vi "Set parameters.vi"(8 "error in (no error)":errorcluster caption="entrée d'erreur (pas d'erreur)", 11 "OWIS_TANGO en entrée":refnum<class "OWIS_TANGO.lvclass">) -> (0 "error out":errorcluster caption="sortie d'erreur", 3 "OWIS_TANGO en sortie":refnum<class "OWIS_TANGO.lvclass">)   [LabVIEW 2020, in "OWIS_TANGO.lvclass"]
uses:
  OWIS_TANGO.lvclass
  C:/dev/TRANCON/Classes/GeneralFunctionality/GeneralFunctionality.lvclass
  C:/dev/TRANCON/Classes/Delay Line/DelayLine.lvclass
  GeneralFunctionality/GeneralFunctionality.lvclass/GeneralFunctionality.ctl
  DelayLineLS4/LS4_parameters.ctl
  Config/Config.lvclass
  DelayLine.lvclass
  GeneralFunctionality/GeneralFunctionality.lvclass
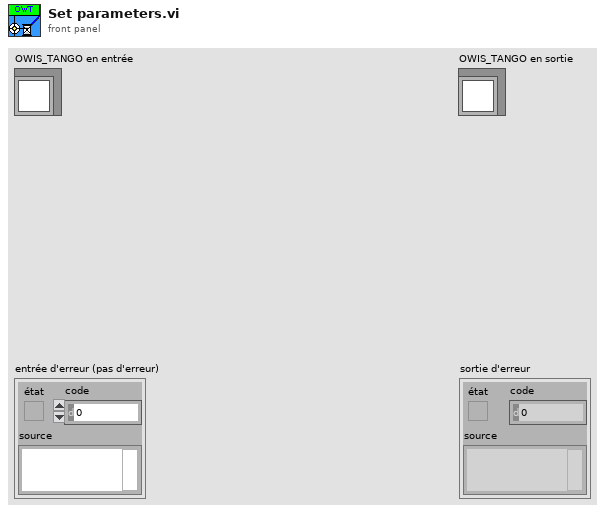
[diagram p1: front panel]
types:
  T1 = typedef "DelayLine.lvclass/LS4_parameters.ctl" = string
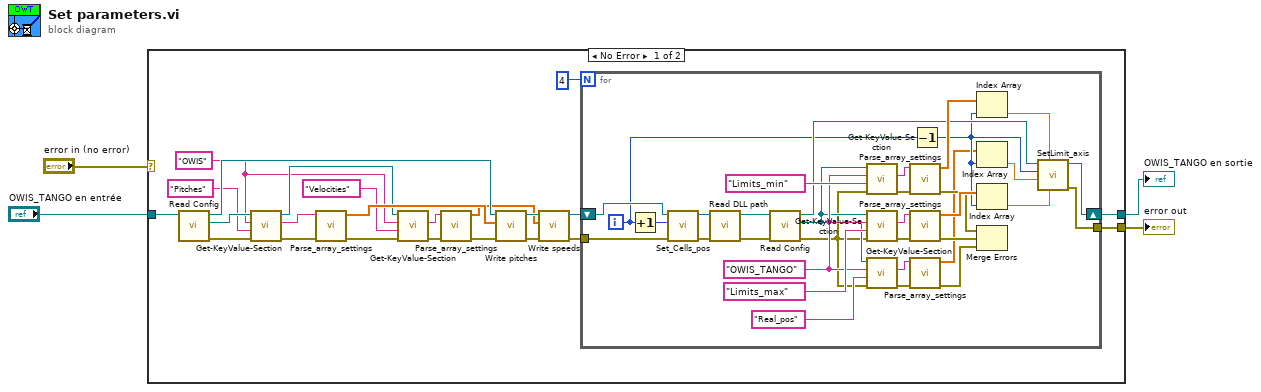
[diagram p0: block diagram]
diagram:
  n1 = case shown="No Error" "error in (no error)" {
    selector: "error in (no error)" -> [_ w62]
    tunnel: [w6 w61] -> w3
    tunnel: "OWIS_TANGO en entrée" -> [w23 w61]
    tunnel: [w7 w62] -> w1
    frame No Error {
      w10 = "OWIS" ("Section")
      n2 = call "Read Config.vi"("GeneralFunctionality en entrée"=w23) -> ("error out"=w19:errorcluster, "Config.lvclass"=w18:refnum<class "Config.lvclass">, "GeneralFunctionality en sortie"=w22:refnum<class "OWIS_TANGO.lvclass">)  [unwired: 8 in]
      n3 = call-dynamic "Get-KeyValue-Section.vi"("error in (no error)"=w19, "Key"="Pitches", "Section"=w10, "Config in"=w18) -> ("error out"=w16:errorcluster, "Value"=w15:string, "Config out"=w14:refnum<class "Config.lvclass">)  [unwired: 5 in]
      n4 = call "Parse_array_settings.vi"("error in (no error)"=w16, "Value"=w15) -> ("error out"=w13:errorcluster, "Array"=w21:dbl[])  [unwired: 8 in]
      n5 = call-dynamic "Get-KeyValue-Section.vi"("error in (no error)"=w13, "Key"="Velocities", "Section"=w10, "Config in"=w14) -> ("error out"=w12:errorcluster, "Value"=w11:string)  [unwired: 5 in, 1 out]
      n6 = call "Parse_array_settings.vi"("error in (no error)"=w12, "Value"=w11) -> ("error out"=w8:errorcluster, "Array"=w20:dbl[])  [unwired: 8 in]
      n7 = call-dynamic "Write pitches.vi"("error in (no error)"=w8, "pitches"=w21, "DelayLine in"=w22) -> ("error out"=w27:errorcluster, "DelayLine out"=w26:refnum<class "OWIS_TANGO.lvclass">)  [unwired: 7 in]
      n8 = call-dynamic "Write speeds.vi"("error in (no error)"=w27, "speeds"=w20, "DelayLine in"=w26) -> ("error out"=w25:errorcluster, "DelayLine out"=w24:refnum<class "OWIS_TANGO.lvclass">)  [unwired: 7 in]
      n9 = for {
        N: 4 -> [_]
        tunnel: w25 -> [w60]
        tunnel: [w33] -> w7
        shift-right: [w32] -> w6
        shift-left: w24 -> [w59]
        i -> [w28]
        w42 = "OWIS_TANGO" ("Section")
        n10 = Increment(x=w28) -> (x+1=w29:i32)
        n11 = call "Set_Cells_pos.vi"("error in (no error)"=w60, "axis"=w29, "DelayLine in"=w59) -> ("error out"=w30:errorcluster, "DelayLine out"=w31:refnum<class "OWIS_TANGO.lvclass">)  [unwired: 7 in]
        n12 = call "Read DLL path.vi"("error in (no error)"=w30, "DelayLine in"=w31) -> ("error out"=w55:errorcluster, "DelayLine out"=w47:refnum<class "OWIS_TANGO.lvclass">)  [unwired: 7 in, 1 out]
        n13 = call "Read Config.vi"("error in (no error)"=w55, "GeneralFunctionality en entrée"=w47) -> ("error out"=w40:errorcluster, "Config.lvclass"=w41:refnum<class "Config.lvclass">, "GeneralFunctionality en sortie"=w46:refnum<class "OWIS_TANGO.lvclass">)  [unwired: 7 in]
        n14 = call-dynamic "Get-KeyValue-Section.vi"("error in (no error)"=w40, "Key"=T1 "Limits_min" ("Section"), "Section"=w42, "Config in"=w41) -> ("error out"=w57:errorcluster, "Value"=w58:string)  [unwired: 5 in, 1 out]
        n15 = call-dynamic "Get-KeyValue-Section.vi"("error in (no error)"=w40, "Key"=T1 "Limits_max" ("Section"), "Section"=w42, "Config in"=w41) -> ("error out"=w53:errorcluster, "Value"=w52:string)  [unwired: 5 in, 1 out]
        n16 = call-dynamic "Get-KeyValue-Section.vi"("error in (no error)"=w40, "Key"="Real_pos", "Section"=w42, "Config in"=w41) -> ("error out"=w36:errorcluster, "Value"=w37:string)  [unwired: 5 in, 1 out]
        n17 = call "Parse_array_settings.vi"("error in (no error)"=w57, "Value"=w58) -> ("error out"=w49:errorcluster, "Array"=w54:dbl[])  [unwired: 8 in]
        n18 = call "Parse_array_settings.vi"("error in (no error)"=w53, "Value"=w52) -> ("error out"=w48:errorcluster, "Array"=w50:dbl[])  [unwired: 8 in]
        n19 = call "Parse_array_settings.vi"("error in (no error)"=w36, "Value"=w37) -> ("error out"=w35:errorcluster, "Array"=w38:dbl[])  [unwired: 8 in]
        n20 = Decrement(x=w28) -> (x-1=w39:i32)
        n21 = Index Array(array=w54, index=w39) -> (element=w45:dbl)
        n22 = Index Array(array=w38, index=w39) -> (element=w34:dbl)
        n23 = Index Array(array=w50, index=w39) -> (element=w44:dbl)
        n24 = Merge Errors(w49, w48, w35) -> ()  [unwired: 1 out]
        n25 = call-dynamic "SetLimit_axis.vi"("max"=w44, "min"=w45, "real pos zero"=w34, "Axis"=w39, "DelayLine in"=w46) -> ("error out"=w33:errorcluster, "DelayLine out"=w32:refnum<class "OWIS_TANGO.lvclass">)  [unwired: 5 in]
      }
    }
    frame Error {
    }
  }
  "error out" <- w1
  "OWIS_TANGO en sortie" <- w3
